vi "Client 1 - Copy2.vi"() -> ()   [LabVIEW 2017]
uses:
  <vilib>/Analysis/Matrix/Datatypes/RealMatrix.ctl
  <vilib>/Analysis/Matrix/NI_Matrix.lvlib
panel:
  out "BYTE WRITE FROM SERVER":i32
  in  "Matrix":T1
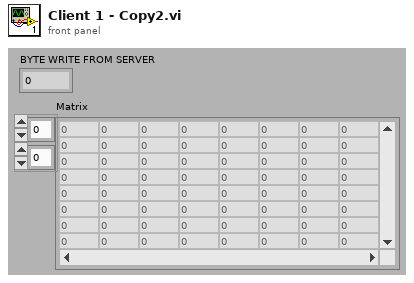
[diagram p1: front panel]
types:
  T1 = typedef "NI_Matrix.lvlib/RealMatrix.ctl" = dbl[][]
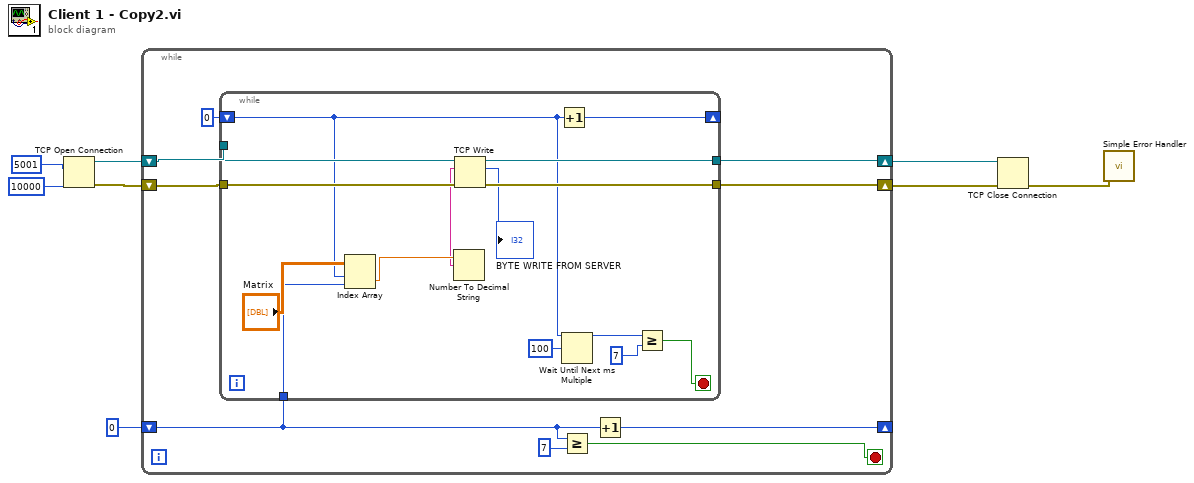
[diagram p0: block diagram]
diagram:
  n1 = TCP Open Connection(remote port or service name=u16 5001, timeout ms (60000)=10000) -> (connection ID=w6:refnum<k5>, error out=w5:errorcluster)  [unwired: 3 in]
  n2 = while {
    shift-right: [w15] -> w3
    shift-left: w6 -> [w17]
    shift-right: [w14] -> w2
    shift-left: w5 -> [w16]
    shift-right: [w12] -> _
    shift-left: 0 -> [w9]
    stop <- w10 stop-if-true
    n3 = while {
      tunnel: w17 -> [w31]
      tunnel: w16 -> [w30]
      tunnel: [w29] -> w15
      tunnel: [w28] -> w14
      shift-right: [w22] -> _
      shift-left: 0 -> [w21]
      tunnel: w9 -> [w18]
      stop <- w19 stop-if-true
      n4 = Index Array(array="Matrix", index (row)=w21, index (col)=w18) -> (element=w25:dbl)
      n5 = Number To Decimal String(number=w25) -> (decimal integer string=w24:string)  [unwired: 1 in]
      n6 = TCP Write(connection ID=w31, data in=w24, error in (no error)=w30) -> (connection ID out=w29:refnum<k5>, bytes written=→"BYTE WRITE FROM SERVER":i32, error out=w28:errorcluster)  [unwired: 1 in]
      n7 = Increment(x=w21) -> (x+1=w22:i32)
      n8 = Wait Until Next ms Multiple(millisecond multiple=u32 100) -> ()  [unwired: 1 out]
      n9 = Greater Or Equal?(x=w21, y=7) -> (x >= y?=w19:bool)
    }
    n10 = Greater Or Equal?(x=w9, y=7) -> (x >= y?=w10:bool)
    n11 = Increment(x=w9) -> (x+1=w12:i32)
  }
  n12 = TCP Close Connection(connection ID=w3, error in (no error)=w2) -> (error out=w4:errorcluster)  [unwired: 1 in, 1 out]
  n13 = call <vilib>:"Simple Error Handler.vi"("error in (no error)"=w4) -> ()  [unwired: 4 in, 5 out]
